vi "Song Element Library To Song Library.vi"(8 "error in (no error)":errorcluster, 11 "MusicElementLibrary":refnum<class "MusicElementLibrary.lvclass">) -> (0 "error out":errorcluster, 3 "SongLibrary out":refnum<class "SongLibrary.lvclass">)   [LabVIEW 2015, in "SongLibrary.lvclass"]
uses:
  SongLibrary.lvclass
  MusicElementLibrary.lvclass
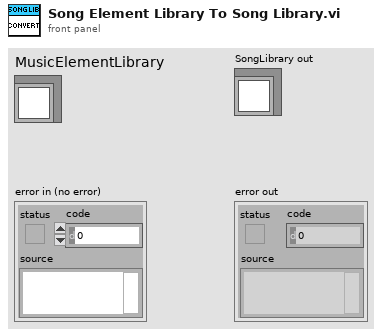
[diagram p1: front panel]
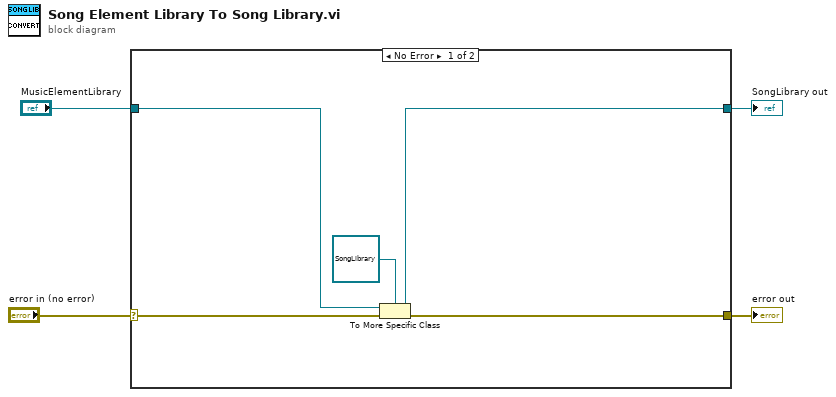
[diagram p0: block diagram]
diagram:
  n1 = case shown="No Error" "error in (no error)" {
    selector: "error in (no error)" -> [w9 w10]
    tunnel: [w5 w10] -> w3
    tunnel: [w6 _] -> w2
    tunnel: "MusicElementLibrary" -> [w7 _]
    frame No Error {
      n2 = To More Specific Class(target class=refnum<class "SongLibrary.lvclass"> refnum ("SongLibrary out 2"), reference=w7, error in=w9) -> (specific class reference=w6:refnum<class "SongLibrary.lvclass">, error out=w5:errorcluster)
    }
    frame Error {
    }
  }
  "error out" <- w3
  "SongLibrary out" <- w2
